vi "EnQueue Actions.vi"(0 "action queue in":refnum<queue>, 5 "actions":string[](array[string]), 7 "data in":string[](array[string]), 11 "error in":errorcluster) -> (4 "action queue out":refnum<queue>, 15 "error out":errorcluster)   [LabVIEW 2016, in "TLB` Template.lvlib" / "Actions.lvlib"]
doc: "Adds multiple elements to the action queue.\n\n<B>Input Parameters</B>\n\n<B>action queue in</B> is a reference to a queue. Use the Create Action Queue function to obtain a queue reference. \n\n<B>action</B> inserted into system.\n\n<B>data in</B> playload into system.\n\n<B>error in</B> describes error conditions that occur before this node runs. This input provides standard error in functionality.\n\n<B>Output Parameters</B>\n\n<B>action queue out</B> returns the reference to the queue unchanged. \n\n<B>error out</B> contains error information. This output provides standard error out functionality."
uses:
  Actions.lvlib
  System Action Element.ctl
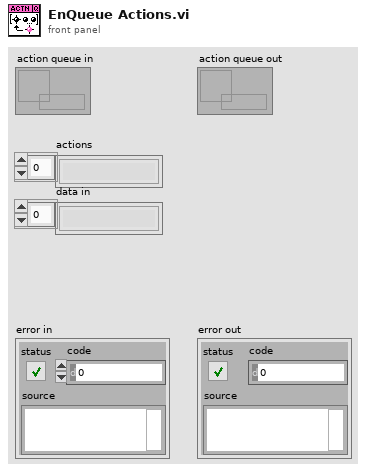
[diagram p1: front panel]
types:
  T1 = typedef "TLB` Template.lvlib/Actions.lvlib/System Action Element.ctl" = cluster{"action":string, "data":string}
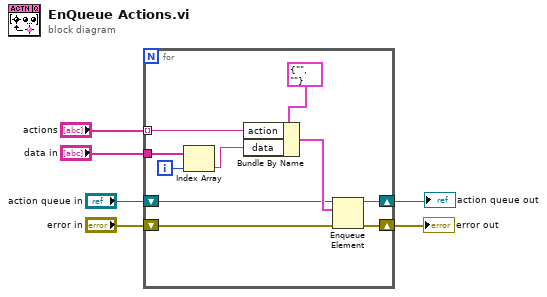
[diagram p0: block diagram]
diagram:
  n1 = for {
    shift-right: [w15] -> w5
    shift-left: "error in" -> [w16]
    shift-right: [w11] -> w3
    shift-left: "action queue in" -> [w12]
    tunnel: "actions" -> [w10] mode=indexing
    tunnel: "data in" -> [w9]
    i -> [w8]
    n2 = Index Array(array=w9, index=w8) -> (element=w7:string)
    n3 = Bundle By Name(cluster=T1 {"action"="", "data"=""} ("System Action Element"), "action"=w10, "data"=w7) -> (w13:T1)
    n4 = Enqueue Element(queue=w12, element=w13, error in (no error)=w16) -> (queue out=w11:refnum<queue>, error out=w15:errorcluster)  [unwired: 1 in, 1 out]
  }
  "error out" <- w5
  "action queue out" <- w3
